vi "mfPSCGenerate.vi"(8 "error in (no error)":errorcluster caption="错误输入（无错误）", 11 "Path":path) -> (0 "error out":errorcluster caption="错误输出", 3 "PSC":cdb[](array[numeric]))   [LabVIEW 2015]
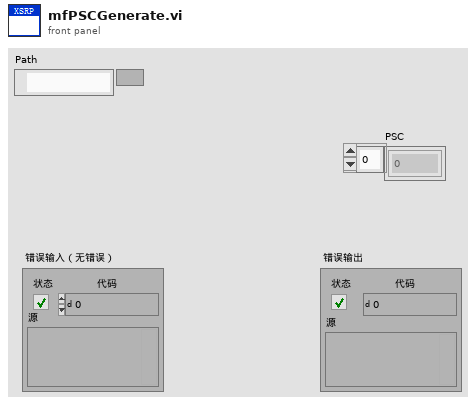
[diagram p1: front panel]
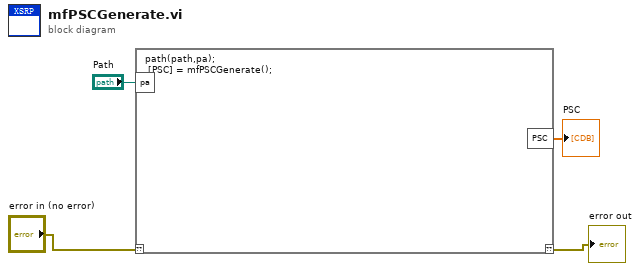
[diagram p0: block diagram]
diagram:
  n1 = script code="path(path,pa);\n [PSC] = mfPSCGenerate();"("??"="error in (no error)", "pa"="Path") -> ("??"=→"error out":errorcluster, "PSC"=→"PSC":cdb[])
